vi "Abbreviate Name.vi"(8 "error in (no error)":errorcluster, 9 "Max Length":i32=6, 10 "Long Name":string) -> (0 "error out":errorcluster, 2 "Abreviated Name":string)   [LabVIEW 2020, in "Method Generation.lvlib" / "Support.lvlib"]
uses:
  Support.lvlib
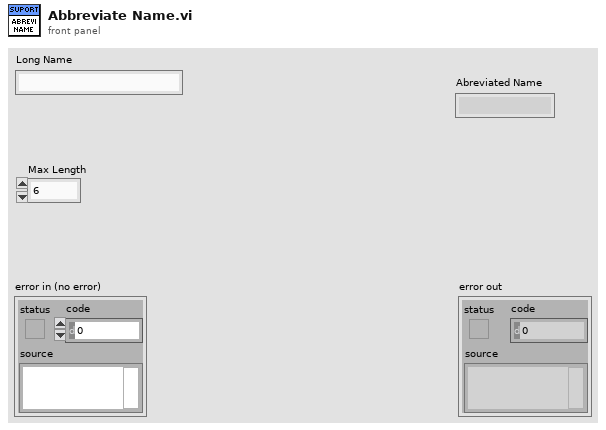
[diagram p1: front panel]
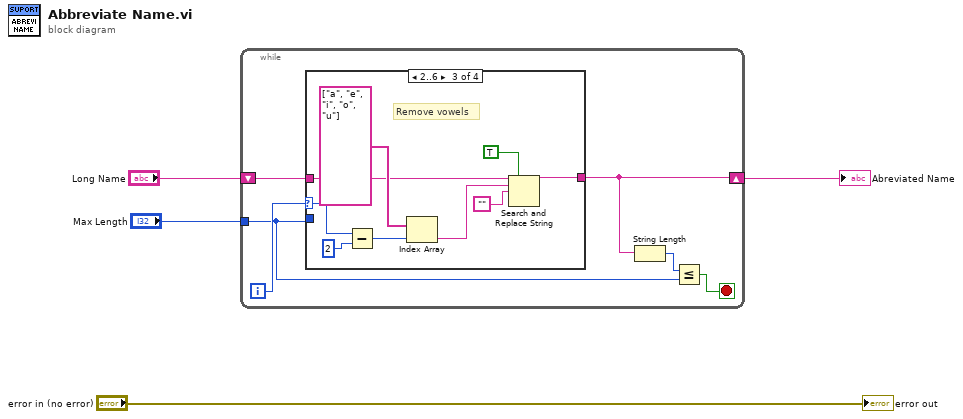
[diagram p0: block diagram]
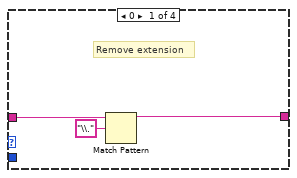
[diagram p2: hidden frame]
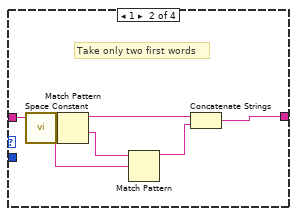
[diagram p3: hidden frame]
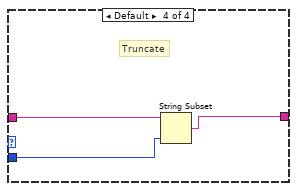
[diagram p4: hidden frame]
diagram:
  n1 = while {
    shift-right: [w6] -> w2
    shift-left: "Long Name" -> [w9]
    tunnel: "Max Length" -> [w5]
    i -> [w10]
    stop <- w7 stop-if-true
    n2 = case shown="2..6" w10 {
      selector: w10 -> [_ _ w27 _]
      tunnel: w9 -> [w13 w19 w24 w31]
      tunnel: [w11 w16 w23 w30] -> w6
      tunnel: w5 -> [_ _ _ w29]
      frame 0 {
        # "Remove extension"
        n3 = Match Pattern(string=w13, regular expression="\\.") -> (before substring=w11:string)  [unwired: 1 in, 3 out]
      }
      frame 1 {
        # "Take only two first words"
        n4 = call <vilib>:"Space Constant.vi"() -> ("String"=w17:string)
        n5 = Match Pattern(string=w19, regular expression=w17) -> (before substring=w18:string, after substring=w14:string)  [unwired: 1 in, 2 out]
        n6 = Match Pattern(string=w14, regular expression=w17) -> (before substring=w15:string)  [unwired: 1 in, 3 out]
        n7 = Concatenate Strings(w18, w15) -> (w16:string)
      }
      frame 2..6 {
        # "Remove vowels"
        n8 = Subtract(x=w27, y=2) -> (x-y=w26:i32)
        n9 = Index Array(array=string[] ["a", "e", "i", "o", "u"], index=w26) -> (element=w21:string)
        n10 = Search and Replace String(replace all?=TRUE ("replace all? (F)"), input string=w24, search string=w21, replace string="") -> (result string=w23:string)  [unwired: 4 in, 3 out]
      }
      frame Default {
        # "Truncate"
        n11 = String Subset(string=w31, length (rest)=w29) -> (substring=w30:string)  [unwired: 1 in]
      }
    }
    n12 = String Length(string=w6) -> (length=w8:i32)
    n13 = Less Or Equal?(x=w8, y=w5) -> (x <= y?=w7:bool)
  }
  "Abreviated Name" <- w2
  "error out" <- "error in (no error)"
